vi "SetSamples.vi"(3 "error in (no error)":errorcluster, 4 "samples":i32, 5 "Task ID":u32) -> (0 "error out":errorcluster, 2 "Task ID":u32)   [LabVIEW 2015]
uses:
  Windows/System32/AdvLvDaq.dll
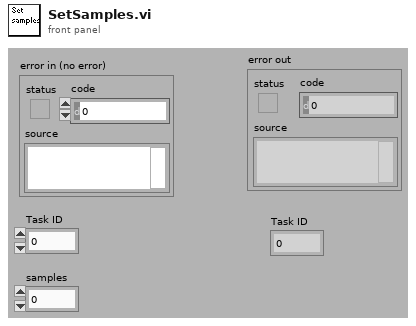
[diagram p1: front panel]
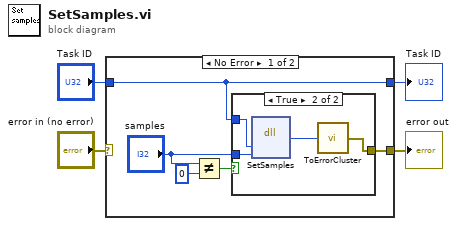
[diagram p0: block diagram]
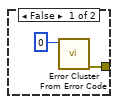
[diagram p2: hidden frame]
diagram:
  n1 = case shown="No Error" "error in (no error)" {
    selector: "error in (no error)" -> [_ w16]
    tunnel: "Task ID" -> [w9 w17]
    tunnel: [w9 w17] -> w2
    tunnel: [w8 w16] -> w1
    frame No Error {
      n2 = Not Equal?(x="samples", y=0) -> (x != y?=w6:bool)
      n3 = case shown="True" w6 {
        tunnel: w9 -> [_ w15]
        tunnel: [w11 w13] -> w8
        tunnel: "samples" -> [_ w12]
        frame False {
          n4 = call <vilib>:"Error Cluster From Error Code.vi"("error code (0)"=0) -> ("error out"=w11:errorcluster)  [unwired: 2 in, 6 out]
        }
        frame True {
          n5 = dll-call lib="C:/Windows/System32/AdvLvDaq.dll" fn="SetSamples"("taskId"=w15, "samples"=w12) -> ("return type"=w14:i32)  [unwired: 5 in, 2 out]
          n6 = call "ToErrorCluster.vi"("error code"=w14) -> ("error out"=w13:errorcluster)
        }
      }
    }
    frame Error {
    }
  }
  "Task ID" <- w2
  "error out" <- w1
